vi "Network Shared Variable Check Reverse.vi"() -> ()   [LabVIEW 2013]
panel:
  in  "stop":bool
  out "PS1Voltage":dbl
  in  "PS2Voltage":dbl
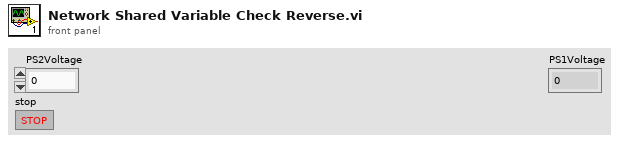
[diagram p1: front panel]
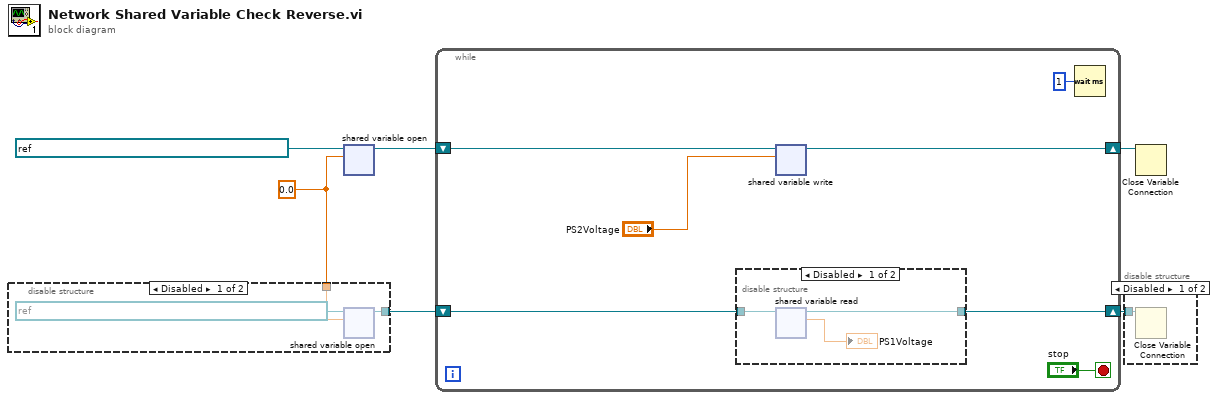
[diagram p0: block diagram]
diagram:
  w2 = 0.0
  n1 = disable-structure shown="Disabled" {
    disable-tunnel: [w9 _] -> w5
    disable-tunnel: w2 -> [w8 _]
    frame Disabled {
      n2 = shared-variable-open(refnum<k21> "ni.var.psp://rt single-board rio/PS Control/PS1Voltage" ("shared variable refnum in"), w8) -> (w9:refnum<k21>)  [unwired: 2 in, 1 out]
    }
    frame Enabled {
    }
  }
  n3 = shared-variable-open(refnum<k21> "ni.var.psp://10.30.189.155/PS Control/PS1CMD" ("shared variable refnum in"), w2) -> (w6:refnum<k21>)  [unwired: 2 in, 1 out]
  n4 = while {
    shift-right: [w11] -> w4
    shift-left: w5 -> [w12]
    shift-right: [w13] -> w3
    shift-left: w6 -> [w14]
    stop <- "stop" stop-if-true
    n5 = disable-structure shown="Disabled" {
      disable-tunnel: w12 -> [w19 _]
      disable-tunnel: [w18 _] -> w11
      frame Disabled {
        n6 = shared-variable-read(w19) -> (w18:refnum<k21>, →"PS1Voltage":dbl)  [unwired: 1 in, 2 out]
      }
      frame Enabled {
      }
    }
    n7 = shared-variable-write(w14, "PS2Voltage") -> (w13:refnum<k21>)  [unwired: 1 in, 1 out]
    n8 = Wait (ms)(milliseconds to wait=u32 1) -> ()  [unwired: 1 out]
  }
  n9 = disable-structure shown="Disabled" {
    disable-tunnel: w4 -> [w20 _]
    frame Disabled {
      n10 = Close Variable Connection(11:w20) -> ()  [unwired: 1 in, 1 out]
    }
    frame Enabled {
    }
  }
  n11 = Close Variable Connection(11:w3) -> ()  [unwired: 1 in, 1 out]
